vi "Select Multiple Files LV 2012 NI Verified.vi"() -> (0 "selected path":path[](array[path]))   [LabVIEW 2018]
panel:
  out "error out":errorcluster
  # "Overview: This example shows how to call a customized file selection dialog allowing to select multiple files\nRequirements: LabVIEW 2012 (or compatible)\nInstructions: \n1. Run the VI\n2. In the Select Multiple Files dialog box, select any files you want, by clicking Ctrl key\n3. Click Thanks LabVIEW!!! to close the dialog box\n4. Selected files indicator will list the paths of the selected files"
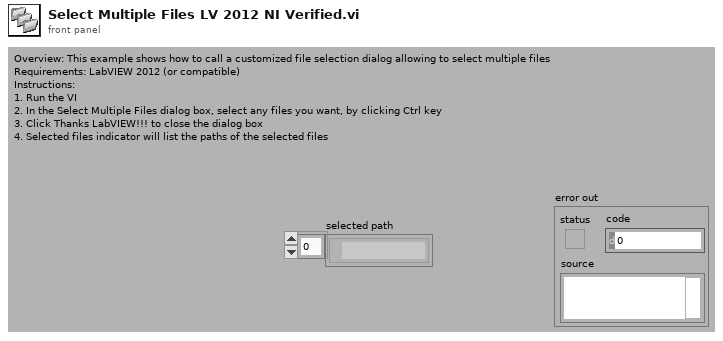
[diagram p1: front panel]
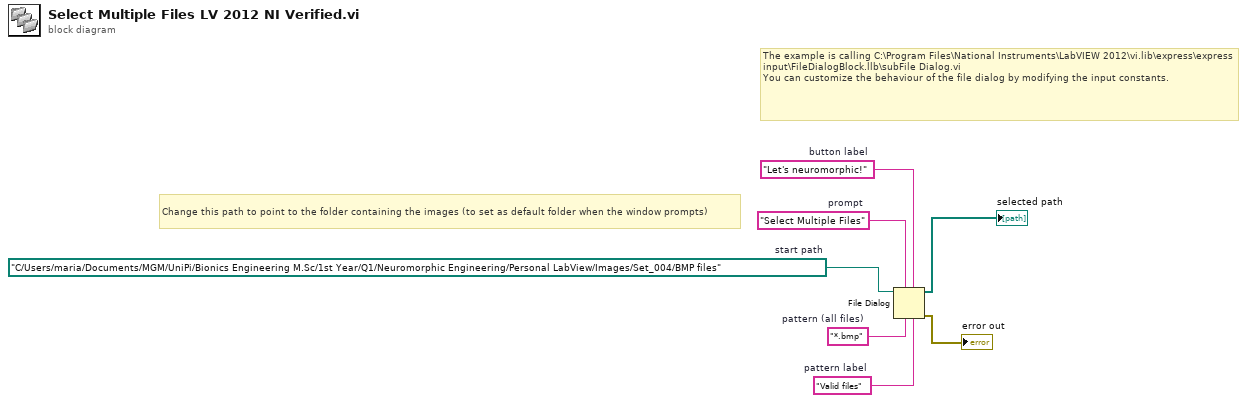
[diagram p0: block diagram]
diagram:
  w1 = "Let's neuromorphic!"  # button label
  w3 = "Select Multiple Files"  # prompt
  w5 = "Valid files"  # pattern label
  w6 = "*.bmp"  # pattern (all files)
  w7 = path "C:/Users/maria/Documents/MGM/UniPi/Bionics Engineering M.Sc/1st Year/Q1/Neuromorphic Engineering/Personal LabView/Images/Set_004/BMP files"  # start path
  # "Change this path to point to the folder containing the images (to set as default folder when the window prompts)"
  # "The example is calling C:\\Program Files\\National Instruments\\LabVIEW 2012\\vi.lib\\express\\express input\\FileDialogBlock.llb\\subFile Dialog.vi\nYou can customize the behaviour of the file dialog by modifying the input constants."
  n1 = File Dialog(4:w5, 5:w1, 6:w6, 7:w3, 11:w7) -> (0:→"error out":errorcluster, 3:→"selected path":path[])  [unwired: 2 in, 2 out]
